vi "Play Selector.vi"() -> (0 "Output Play":T1)   [LabVIEW 2014]
uses:
  Autonomous Play Definition.ctl
  Autonomous Commands/Autonomous Command Names.ctl
  <vilib>/Rock Robotics/Network Tables/SD Read String.vi
  Global Variables/Autonomous Play Globals.vi
panel:
  out "error out":errorcluster
  out "rest of the binary string":string
  out "File Name of Play":string
  # "Add as many plays \nas needed or are supported\nby the number of bits in\nplay selector\n\nRemember Ryan wants \nno less than 32 \nautonomous plays\n\nREMEMBER TO SAVE ALL \nVALUES AS DEFAULT \nEVERYTIME YOU MAKE \nCHANGES TO PLAYS"
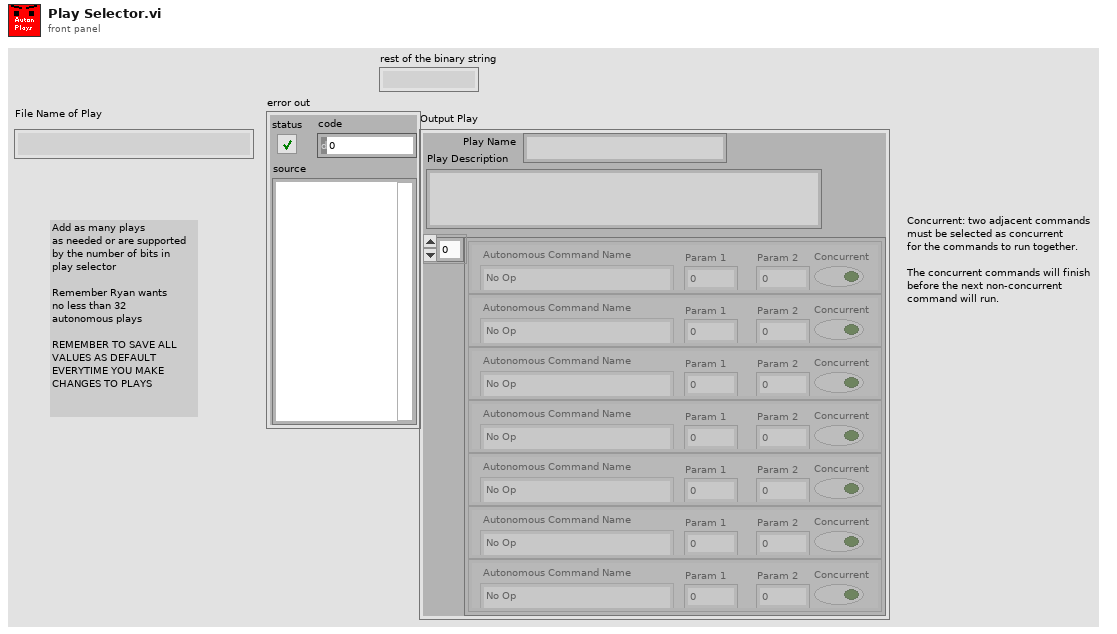
[diagram p1: front panel]
types:
  T1 = typedef "Autonomous Play Definition.ctl" = cluster{"Play Name":string, "Command List":cluster{"Param 1":dbl, "Param 2":dbl, "Autonomous Command Name":T2, "Concurrent":bool}[], "Play Description":string}
  T2 = typedef "Autonomous Command Names.ctl" = enum16{"No Op", "Drive Distance Robot", "Drive Time Robot", "Translate Distance Robot", "Translate Time Robot", "Drive Distance Field", "Drive Time Field", "Translate Distance Field", "Translate Time Field", "Rotate Robot", "Set Initial Gyro Value", "Lifter to Setpoint", "Wait", "Do Not use", "Drive Distance Field (Gyro Hold)", "Translate Distance Field (Gyro Hold)", "Can", "Grabber", "Drive Distance Field (Sensor Stop, Gyro Hold)", "Move Direction Field (Gyro Hold)", "Rotate Robot 90 about Tote", "Reset Gyro", "Find Tote", "Get Tote Into Robot", "Lower Can Grabber"}
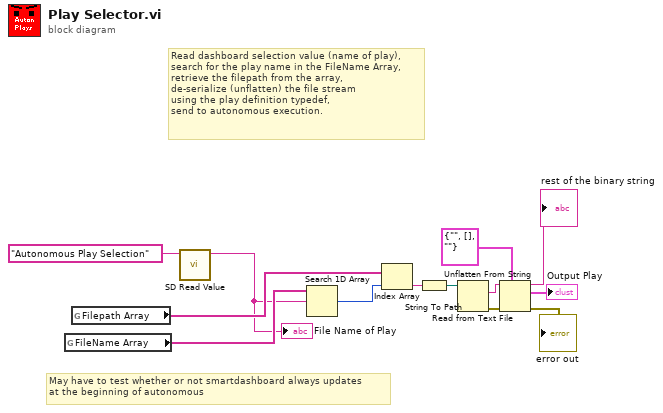
[diagram p0: block diagram]
diagram:
  # "May have to test whether or not smartdashboard always updates\nat the beginning of autonomous"
  # "Read dashboard selection value (name of play), \nsearch for the play name in the FileName Array,\nretrieve the filepath from the array,\nde-serialize (unflatten) the file stream\nusing the play definition typedef, \nsend to autonomous execution."
  n1 = global read "Autonomous Play Globals.vi" "FileName Array"() -> (w13:string[])
  n2 = global read "Autonomous Play Globals.vi" "Filepath Array"() -> (w12:string[])
  n3 = call-poly <vilib>:"SD Read Value.vi"("Name"="Autonomous Play Selection") -> ("String"=w4:string)  [unwired: 8 in, 2 out]
  "File Name of Play" <- w4
  n4 = Search 1D Array(1D array=w13, element=w4) -> (index of element=w11:i32)  [unwired: 1 in]
  n5 = Index Array(array=w12, index=w11) -> (element=w10:string)
  n6 = String To Path(string=w10) -> (path=w9:path)
  n7 = Read from Text File(file (use dialog)=w9) -> (text=w8:string, error out=w1:errorcluster)  [unwired: 3 in, 2 out]
  n8 = Unflatten From String(type=T1 {"Play Name"="", "Command List"=[], "Play Description"=""} ("Play 1"), binary string=w8, error in (no error)=w1) -> (rest of the binary string=→"rest of the binary string":string, value=→"Output Play":T1, error out=→"error out":errorcluster)  [unwired: 2 in]
